vi "核查数据发送(子VI).vi"(8 "错误输入":errorcluster) -> (0 "错误输出":errorcluster)   [LabVIEW 2016, in "数据传输系统.lvlib"]
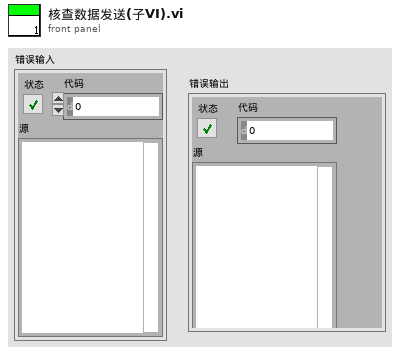
[diagram p1: front panel]
types:
  T1 = enum16{"质控数据", "操作日志", "仪器参数", "系统状态", "运行模式", "测量周期", "超标留样", "报警信息", "环境参数"}
  T2 = enum16{"空白测试", "跨度核查", "标样核查", "加标回收", "平行样", "集成干预"}
  T3 = cluster{"氨氮零点核查索引起始时间":string, "总磷零点核查索引起始时间":string, "总氮零点核查索引起始时间":string, "CODMn零点核查索引起始时间":string, "CODCr零点核查索引起始时间":string, "亚硝酸盐零点核查索引起始时间":string, "硫化物零点核查索引起始时间":string, "ORP零点核查索引起始时间":string}
  T4 = cluster{"[0]":string, "[1]":string, "[2]":string, "[3]":string, "[4]":string, "[5]":string, "[6]":string, "[7]":string}
  T5 = cluster{"PH":string[][], "CODCr":string[][], "氨氮":string[][], "CODMn":string[][], "总氮":string[][], "总磷":string[][], "电导率":string[][], "水温":string[][], "DO":string[][], "浊度":string[][], "叶绿素":string[][], "藻密度":string[][], "铜":string[][], "盐度":string[][], "水位":string[][], "流速":string[][], "瞬时流量":string[][], "累积流量":string[][], "亚硝酸盐":string[][], "硫化物":string[][], "ORP":string[][], "铅":string[][], "镉":string[][], "锌":string[][], "镍":string[][], "锰":string[][], "汞":string[][], "气温":string[][], "气压":string[][], "风速":string[][], "风向":string[][]}
  T6 = cluster{"氨氮跨度核查索引起始时间":string, "总磷跨度核查索引起始时间":string, "总氮跨度核查索引起始时间":string, "CODMn跨度核查索引起始时间":string, "CODCr跨度核查索引起始时间":string, "亚硝酸盐跨度核查索引起始时间":string, "硫化物跨度核查索引起始时间":string, "ORP跨度核查索引起始时间":string}
  T7 = cluster{"氨氮标样核查索引起始时间":string, "总磷标样核查索引起始时间":string, "总氮标样核查索引起始时间":string, "CODMn标样核查索引起始时间":string, "CODCr标样核查索引起始时间":string, "DO标样核查索引起始时间":string, "PH标样核查索引起始时间":string, "比电导率标样核查索引起始时间":string, "水温标样核查索引起始时间":string, "浊度标样核查索引起始时间":string, "叶绿素a标样核查索引起始时间":string, "藻密度标样核查索引起始时间":string, "亚硝酸盐标样核查索引起始时间":string, "硫化物标样核查索引起始时间":string, "ORP标样核查索引起始时间":string}
  T8 = cluster{"[0]":string, "[1]":string, "[2]":string, "[3]":string, "[4]":string, "[5]":string, "[6]":string, "[7]":string, "[8]":string, "[9]":string, "[10]":string, "[11]":string, "[12]":string, "[13]":string, "[14]":string}
  T9 = cluster{"氨氮加标回收索引起始时间":string, "总磷加标回收索引起始时间":string, "总氮加标回收索引起始时间":string, "CODMn加标回收索引起始时间":string, "CODCr加标回收索引起始时间":string}
  T10 = cluster{"[0]":string, "[1]":string, "[2]":string, "[3]":string, "[4]":string}
  T11 = cluster{"氨氮平行样索引起始时间":string, "总磷平行样索引起始时间":string, "总氮平行样索引起始时间":string, "CODMn平行样索引起始时间":string, "CODCr平行样索引起始时间":string}
  T12 = cluster{"氨氮集成干预索引起始时间":string, "总磷集成干预索引起始时间":string, "总氮集成干预索引起始时间":string, "CODMn集成干预索引起始时间":string, "CODCr集成干预索引起始时间":string, "DO集成干预索引起始时间":string, "PH集成干预索引起始时间":string, "比电导率集成干预索引起始时间":string, "水温集成干预索引起始时间":string, "浊度集成干预索引起始时间":string, "叶绿素a集成干预索引起始时间":string, "藻密度集成干预索引起始时间":string, "亚硝酸盐集成干预索引起始时间":string, "硫化物集成干预索引起始时间":string, "ORP集成干预索引起始时间":string}
  T13 = cluster{"氨氮仪器日志索引起始时间":string, "总磷仪器日志索引起始时间":string, "总氮仪器日志索引起始时间":string, "CODMn仪器日志索引起始时间":string, "CODCr仪器日志索引起始时间":string, "系统仪器日志索引起始时间":string}
  T14 = cluster{"[0]":string, "[1]":string, "[2]":string, "[3]":string, "[4]":string, "[5]":string}
  T15 = cluster{"氨氮仪器参数索引起始时间":string, "总磷仪器参数索引起始时间":string, "总氮仪器参数索引起始时间":string, "CODMn仪器参数索引起始时间":string, "CODCr仪器参数索引起始时间":string, "DO仪器参数索引起始时间":string, "PH仪器参数索引起始时间":string, "比电导率仪器参数索引起始时间":string, "水温仪器参数索引起始时间":string, "浊度仪器参数索引起始时间":string, "叶绿素a仪器参数索引起始时间":string, "藻密度仪器参数索引起始时间":string, "ORP仪器参数索引起始时间":string}
  T16 = cluster{"[0]":string, "[1]":string, "[2]":string, "[3]":string, "[4]":string, "[5]":string, "[6]":string, "[7]":string, "[8]":string, "[9]":string, "[10]":string, "[11]":string, "[12]":string}
  T17 = cluster{"氨氮报警信息索引起始时间":string, "总磷报警信息索引起始时间":string, "总氮报警信息索引起始时间":string, "CODMn报警信息索引起始时间":string, "CODCr报警信息索引起始时间":string, "DO报警信息索引起始时间":string, "PH报警信息索引起始时间":string, "比电导率报警信息索引起始时间":string, "水温报警信息索引起始时间":string, "浊度报警信息索引起始时间":string, "叶绿素报警信息索引起始时间":string, "系统报警信息索引起始时间":string}
  T18 = cluster{"[0]":string, "[1]":string, "[2]":string, "[3]":string, "[4]":string, "[5]":string, "[6]":string, "[7]":string, "[8]":string, "[9]":string, "[10]":string, "[11]":string}
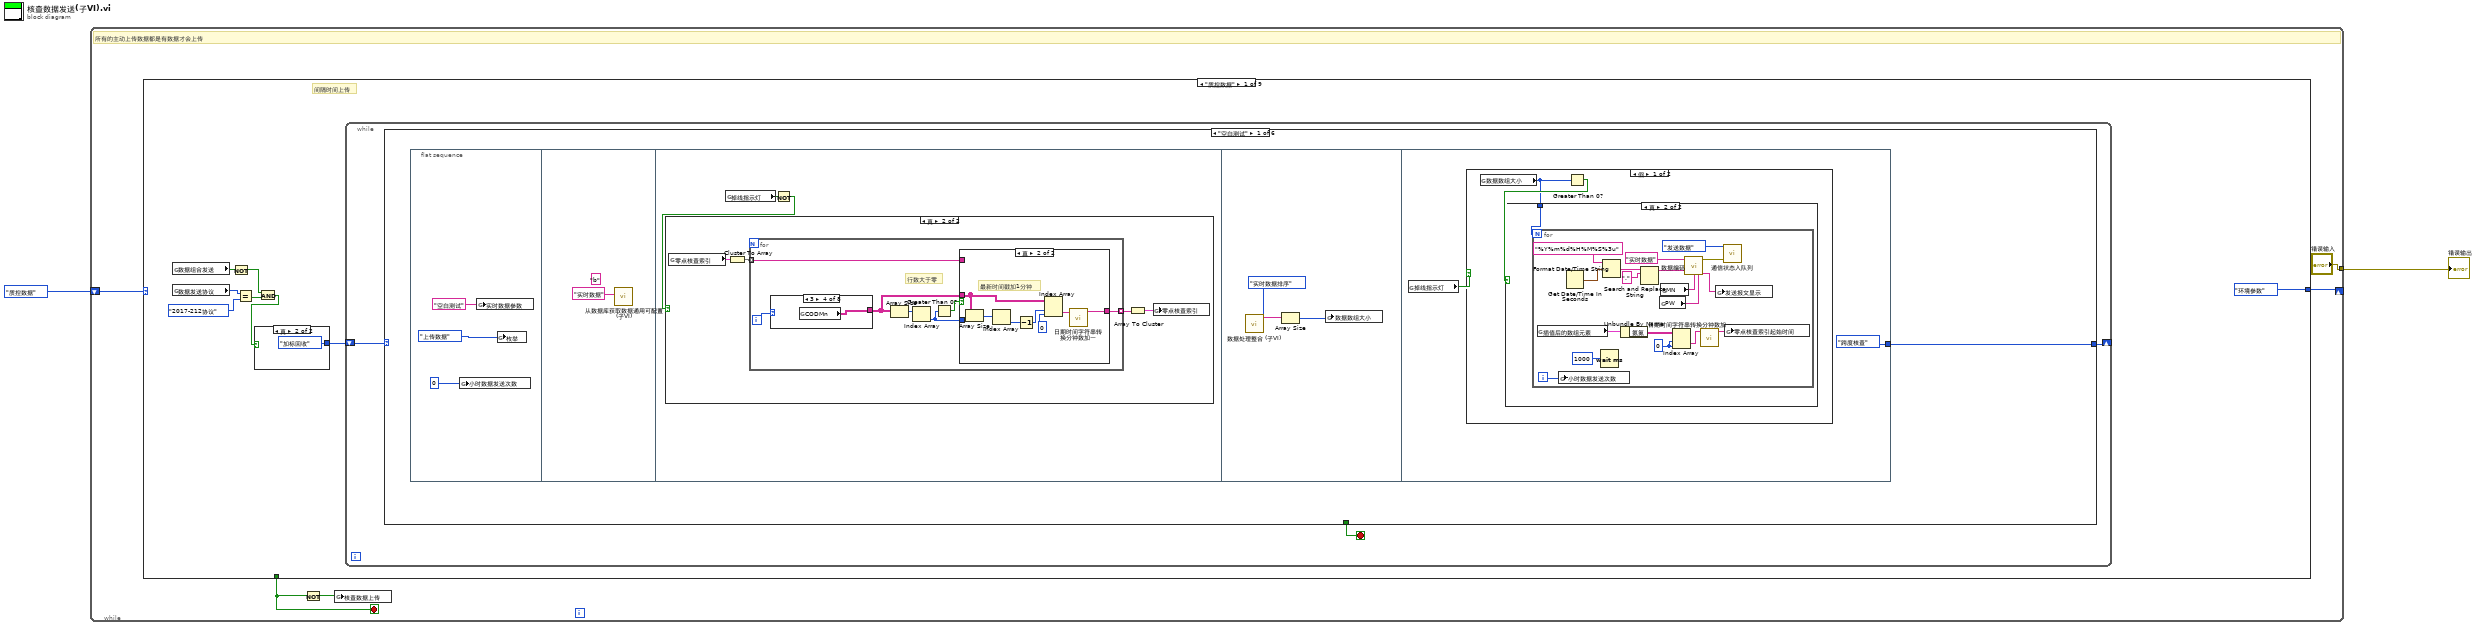
[diagram p0: block diagram]
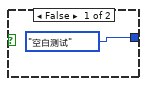
[diagram p2: hidden frame]
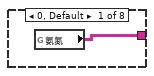
[diagram p4: hidden frame]
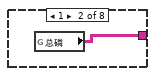
[diagram p5: hidden frame]
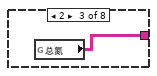
[diagram p6: hidden frame]
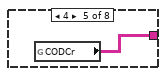
[diagram p7: hidden frame]
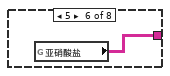
[diagram p8: hidden frame]
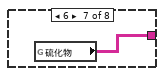
[diagram p9: hidden frame]
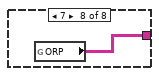
[diagram p10: hidden frame]
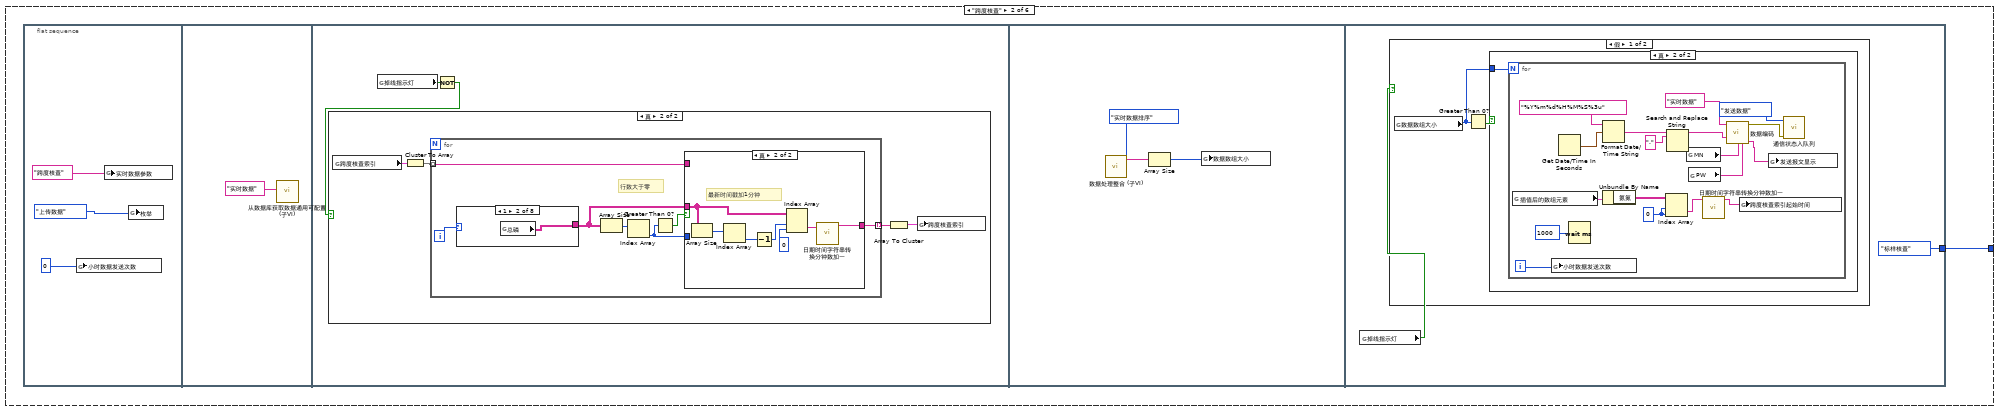
[diagram p14: hidden frame]
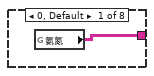
[diagram p16: hidden frame]
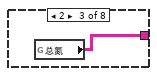
[diagram p17: hidden frame]
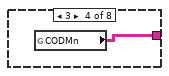
[diagram p18: hidden frame]
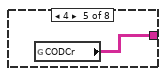
[diagram p19: hidden frame]
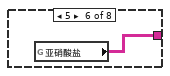
[diagram p20: hidden frame]
diagram:
  n1 = while "While循环" {
    shift-right: [w6] -> _
    shift-left: T1."质控数据" -> [w7]
    tunnel: ["错误输入"] -> w1
    stop <- w4 stop-if-true
    # "所有的主动上传数据都是有数据才会上传"
    n2 = case shown="\"质控数据\"" w7 {
      tunnel: [T1."环境参数" T1."仪器参数" T1."系统状态" T1."运行模式" T1."测量周期" T1."超标留样" T1."报警信息" T1."环境参数" T1."环境参数"] -> w6
      tunnel: [_ _ _ _ _ _ _ _ TRUE] -> w4
      frame "质控数据" {
        # "间隔时间上传"
        n3 = global read "断电保存全局.vi" "数据组合发送"() -> (w10:bool)
        n4 = global read "断电保存全局.vi" "数据发送协议"() -> (w13:enum16{"2005-212协议", "2017-212协议"})
        n5 = Not(x=w10) -> (.not. x?=w9:bool)
        n6 = Equal?(x=w13, y=enum16{"2005-212协议", "2017-212协议"}."2017-212协议" ("数据发送协议")) -> (x = y?=w11:bool)
        n7 = And(x=w9, y=w11) -> (x .and. y?=w8:bool)
        n8 = case shown="真" w8 {
          tunnel: [T2."空白测试" T2."加标回收"] -> w15
          frame False {
          }
          frame True {
          }
        }
        n9 = while {
          shift-right: [w18] -> _
          shift-left: w15 -> [w19]
          stop <- w20 stop-if-true
          n10 = case shown="\"空白测试\"" w19 {
            tunnel: [_ _ _ _ _ TRUE] -> w20
            tunnel: [w21 w81 w141 w208 w267 w319] -> w18
            frame "空白测试" {
              n11 = flat-sequence {
                tunnel: [T2."跨度核查"] -> w21
                frame #0 {
                  n12 = global write "全局 小时数据发送次数.vi" "小时数据发送次数"(0 ("小时数据发送次数")) -> ()
                  n13 = global write "全局 实时数据参数.vi" "实时数据参数"("空白测试") -> ()
                  n14 = global write "全局1.vi" "枚举"(enum16{"返回请求应答", "上传数据", "返回执行结果"}."上传数据" ("枚举")) -> ()
                }
                frame #1 {
                  (unwired) "b" ("列队名（唯一）")
                  n15 = call "从数据库获取数据通用可配置(子VI).vi"("table输入"="实时数据" ("新元素/子数组")) -> ()  [unwired: 9 in, 2 out]
                }
                frame #2 {
                  n16 = global read "全局 数据发送重叠.vi" "掉线指示灯"() -> (w27:bool)
                  n17 = Not(x=w27) -> (.not. x?=w26:bool)
                  n18 = case shown="真" w26 {
                    frame False {
                    }
                    frame True {
                      n19 = global read "全局 时间2.vi" "零点核查索引"() -> (w31:T3)
                      n20 = Cluster To Array(cluster=w31) -> (array=w30:string[])
                      n21 = for {
                        tunnel: [w33] -> w29 mode=indexing
                        tunnel: w30 -> [w32] mode=indexing
                        i -> [w34]
                        # "行数大于零"
                        n22 = case shown="3" w34 {
                          tunnel: [w39 w40 w41 w42 w43 w44 w45 w46] -> w35
                          frame 0, Default {
                            n23 = global read "全局 所有参数.vi" "氨氮"() -> (w39:string[][])
                          }
                          frame 1 {
                            n24 = global read "全局 所有参数.vi" "总磷"() -> (w40:string[][])
                          }
                          frame 2 {
                            n25 = global read "全局 所有参数.vi" "总氮"() -> (w41:string[][])
                          }
                          frame 3 {
                            n26 = global read "全局 所有参数.vi" "CODMn"() -> (w42:string[][])
                          }
                          frame 4 {
                            n27 = global read "全局 所有参数.vi" "CODCr"() -> (w43:string[][])
                          }
                          frame 5 {
                            n28 = global read "全局 所有参数.vi" "亚硝酸盐"() -> (w44:string[][])
                          }
                          frame 6 {
                            n29 = global read "全局 所有参数.vi" "硫化物"() -> (w45:string[][])
                          }
                          frame 7 {
                            n30 = global read "全局 所有参数.vi" "ORP"() -> (w46:string[][])
                          }
                        }
                        n31 = Array Size(array=w35) -> (size(s)=w37:i32[])
                        n32 = Index Array(array=w37) -> (element=w36:i32)  [unwired: 1 in]
                        n33 = Greater Than 0?(x=w36) -> (x > 0?=w38:bool)
                        n34 = case shown="真" w38 {
                          tunnel: w36 -> [_ _]
                          tunnel: w35 -> [_ w50]
                          tunnel: [w47 w48] -> w33
                          tunnel: w32 -> [w47 _]
                          frame False {
                          }
                          frame True {
                            # "最新时间戳加1分钟"
                            n35 = Array Size(array=w50) -> (size(s)=w53:i32[])
                            n36 = Index Array(array=w53) -> (element=w52:i32)  [unwired: 1 in]
                            n37 = Decrement(x=w52) -> (x-1=w51:i32)
                            n38 = Index Array(array=w50, index (row)=w51, index (col)=0 ("禁用的索引 (列)")) -> (element=w54:string)
                            n39 = call "日期时间字符串转换分钟数加一.vi"("data[0]"=w54) -> ("日期/时间字符串"=w48:string)  [unwired: 10 in]
                          }
                        }
                      }
                      n40 = Array To Cluster(array=w29) -> (cluster=w28:T4)
                      n41 = global write "全局 时间2.vi" "零点核查索引"(w28) -> ()
                    }
                  }
                }
                frame #3 {
                  n42 = call "数据处理整合 (子VI).vi"("枚举"=enum16{"实时数据排序", "小时数据排序"}."实时数据排序") -> ("已排序的数组"=w57:string[])  [unwired: 10 in]
                  n43 = Array Size(array=w57) -> (size(s)=w56:i32)
                  n44 = global write "全局 数据数组大小.vi" "数据数组大小"(w56) -> ()
                }
                frame #4 {
                  n45 = global read "全局 数据发送重叠.vi" "掉线指示灯"() -> (w59:bool)
                  n46 = case shown="假" w59 {
                    frame False {
                      n47 = global read "全局 数据数组大小.vi" "数据数组大小"() -> (w60:i32)
                      n48 = Greater Than 0?(x=w60) -> (x > 0?=w61:bool)
                      n49 = case shown="真" w61 {
                        tunnel: w60 -> [_ w62]
                        frame False {
                        }
                        frame True {
                          n50 = for {
                            N: w62 -> [_]
                            i -> [w63]
                            w75 = 0 ("禁用的索引 (列)")
                            n51 = global read "插值后的新数组.vi" "插值后的数组元素"() -> (w79:T5)
                            n52 = global write "全局 小时数据发送次数.vi" "小时数据发送次数"(w63) -> ()
                            n53 = Get Date/Time In Seconds() -> (seconds since 1Jan1904=w67:timestamp)
                            n54 = Wait (ms)(milliseconds to wait=u32 1000 ("等待时间（毫秒）")) -> ()  [unwired: 1 out]
                            n55 = Format Date/Time String(time format string (%c)="%Y%m%d%H%M%S%3u" ("时间格式字符串(%c)"), seconds (now)=w67) -> (date/time string=w66:string)  [unwired: 1 in]
                            n56 = Unbundle By Name(w79) -> ("氨氮"=w78:string[][])
                            n57 = Search and Replace String(input string=w66, search string="." ("搜索字符串")) -> (result string=w64:string)  [unwired: 6 in, 3 out]
                            n58 = global read "断电保存全局.vi" "PW"() -> (w71:string)
                            n59 = global read "断电保存全局.vi" "MN"() -> (w72:string)
                            n60 = Index Array(array=w78, index (row)=w75, index (col)=w75) -> (element=w77:string)
                            n61 = call "数据编码.vi"("table输入"="实时数据" ("新元素/子数组"), "QN"=w64, "MN"=w72, "PW"=w71) -> ("错误常量"=w70:errorcluster, "通讯包字符串"=w74:string)  [unwired: 10 in]
                            n62 = call "日期时间字符串转换分钟数加一.vi"("data[0]"=w77) -> ("日期/时间字符串"=w76:string)  [unwired: 10 in]
                            n63 = global write "全局1.vi" "发送报文显示"(w74) -> ()
                            n64 = call "通信状态入队列.vi"("错误输入（无错误）"=w70, "枚举"=enum16{"打开连接", "发送数据", "读取数据", "数据处理", "关闭连接"}."发送数据") -> ()  [unwired: 9 in, 1 out]
                            n65 = global write "全局 时间2.vi" "零点核查索引起始时间"(w76) -> ()
                          }
                        }
                      }
                    }
                    frame True {
                    }
                  }
                }
              }
            }
            frame "跨度核查" {
              n66 = flat-sequence {
                tunnel: [T2."标样核查"] -> w81
                frame #0 {
                  n67 = global write "全局 小时数据发送次数.vi" "小时数据发送次数"(0 ("小时数据发送次数")) -> ()
                  n68 = global write "全局 实时数据参数.vi" "实时数据参数"("跨度核查") -> ()
                  n69 = global write "全局1.vi" "枚举"(enum16{"返回请求应答", "上传数据", "返回执行结果"}."上传数据" ("枚举")) -> ()
                }
                frame #1 {
                  n70 = call "从数据库获取数据通用可配置(子VI).vi"("table输入"="实时数据" ("新元素/子数组")) -> ()  [unwired: 9 in, 2 out]
                }
                frame #2 {
                  n71 = global read "全局 数据发送重叠.vi" "掉线指示灯"() -> (w87:bool)
                  n72 = Not(x=w87) -> (.not. x?=w86:bool)
                  n73 = case shown="真" w86 {
                    frame False {
                    }
                    frame True {
                      n74 = global read "全局 时间2.vi" "跨度核查索引"() -> (w91:T6)
                      n75 = Cluster To Array(cluster=w91) -> (array=w90:string[])
                      n76 = for {
                        tunnel: [w93] -> w89 mode=indexing
                        tunnel: w90 -> [w92] mode=indexing
                        i -> [w94]
                        # "行数大于零"
                        n77 = case shown="1" w94 {
                          tunnel: [w99 w100 w101 w102 w103 w104 w105 w106] -> w95
                          frame 0, Default {
                            n78 = global read "全局 所有参数.vi" "氨氮"() -> (w99:string[][])
                          }
                          frame 1 {
                            n79 = global read "全局 所有参数.vi" "总磷"() -> (w100:string[][])
                          }
                          frame 2 {
                            n80 = global read "全局 所有参数.vi" "总氮"() -> (w101:string[][])
                          }
                          frame 3 {
                            n81 = global read "全局 所有参数.vi" "CODMn"() -> (w102:string[][])
                          }
                          frame 4 {
                            n82 = global read "全局 所有参数.vi" "CODCr"() -> (w103:string[][])
                          }
                          frame 5 {
                            n83 = global read "全局 所有参数.vi" "亚硝酸盐"() -> (w104:string[][])
                          }
                          frame 6 {
                            n84 = global read "全局 所有参数.vi" "硫化物"() -> (w105:string[][])
                          }
                          frame 7 {
                            n85 = global read "全局 所有参数.vi" "ORP"() -> (w106:string[][])
                          }
                        }
                        n86 = Array Size(array=w95) -> (size(s)=w97:i32[])
                        n87 = Index Array(array=w97) -> (element=w96:i32)  [unwired: 1 in]
                        n88 = Greater Than 0?(x=w96) -> (x > 0?=w98:bool)
                        n89 = case shown="真" w98 {
                          tunnel: w96 -> [_ _]
                          tunnel: w95 -> [_ w110]
                          tunnel: [w107 w108] -> w93
                          tunnel: w92 -> [w107 _]
                          frame False {
                          }
                          frame True {
                            # "最新时间戳加1分钟"
                            n90 = Array Size(array=w110) -> (size(s)=w113:i32[])
                            n91 = Index Array(array=w113) -> (element=w112:i32)  [unwired: 1 in]
                            n92 = Decrement(x=w112) -> (x-1=w111:i32)
                            n93 = Index Array(array=w110, index (row)=w111, index (col)=0 ("禁用的索引 (列)")) -> (element=w114:string)
                            n94 = call "日期时间字符串转换分钟数加一.vi"("data[0]"=w114) -> ("日期/时间字符串"=w108:string)  [unwired: 10 in]
                          }
                        }
                      }
                      n95 = Array To Cluster(array=w89) -> (cluster=w88:T4)
                      n96 = global write "全局 时间2.vi" "跨度核查索引"(w88) -> ()
                    }
                  }
                }
                frame #3 {
                  n97 = call "数据处理整合 (子VI).vi"("枚举"=enum16{"实时数据排序", "小时数据排序"}."实时数据排序") -> ("已排序的数组"=w117:string[])  [unwired: 10 in]
                  n98 = Array Size(array=w117) -> (size(s)=w116:i32)
                  n99 = global write "全局 数据数组大小.vi" "数据数组大小"(w116) -> ()
                }
                frame #4 {
                  n100 = global read "全局 数据发送重叠.vi" "掉线指示灯"() -> (w119:bool)
                  n101 = case shown="假" w119 {
                    frame False {
                      n102 = global read "全局 数据数组大小.vi" "数据数组大小"() -> (w120:i32)
                      n103 = Greater Than 0?(x=w120) -> (x > 0?=w121:bool)
                      n104 = case shown="真" w121 {
                        tunnel: w120 -> [_ w122]
                        frame False {
                        }
                        frame True {
                          n105 = for {
                            N: w122 -> [_]
                            i -> [w123]
                            w135 = 0 ("禁用的索引 (列)")
                            n106 = global read "插值后的新数组.vi" "插值后的数组元素"() -> (w139:T5)
                            n107 = global write "全局 小时数据发送次数.vi" "小时数据发送次数"(w123) -> ()
                            n108 = Get Date/Time In Seconds() -> (seconds since 1Jan1904=w127:timestamp)
                            n109 = Wait (ms)(milliseconds to wait=u32 1000 ("等待时间（毫秒）")) -> ()  [unwired: 1 out]
                            n110 = Format Date/Time String(time format string (%c)="%Y%m%d%H%M%S%3u" ("时间格式字符串(%c)"), seconds (now)=w127) -> (date/time string=w126:string)  [unwired: 1 in]
                            n111 = Unbundle By Name(w139) -> ("氨氮"=w138:string[][])
                            n112 = Index Array(array=w138, index (row)=w135, index (col)=w135) -> (element=w137:string)
                            n113 = Search and Replace String(input string=w126, search string="." ("搜索字符串")) -> (result string=w124:string)  [unwired: 6 in, 3 out]
                            n114 = global read "断电保存全局.vi" "MN"() -> (w133:string)
                            n115 = global read "断电保存全局.vi" "PW"() -> (w132:string)
                            n116 = call "日期时间字符串转换分钟数加一.vi"("data[0]"=w137) -> ("日期/时间字符串"=w136:string)  [unwired: 10 in]
                            n117 = call "数据编码.vi"("table输入"="实时数据" ("新元素/子数组"), "QN"=w124, "MN"=w133, "PW"=w132) -> ("错误常量"=w130:errorcluster, "通讯包字符串"=w131:string)  [unwired: 10 in]
                            n118 = global write "全局 时间2.vi" "跨度核查索引起始时间"(w136) -> ()
                            n119 = global write "全局1.vi" "发送报文显示"(w131) -> ()
                            n120 = call "通信状态入队列.vi"("错误输入（无错误）"=w130, "枚举"=enum16{"打开连接", "发送数据", "读取数据", "数据处理", "关闭连接"}."发送数据") -> ()  [unwired: 9 in, 1 out]
                          }
                        }
                      }
                    }
                    frame True {
                    }
                  }
                }
              }
            }
            frame "标样核查" {
              n121 = flat-sequence {
                tunnel: [T2."加标回收"] -> w141
                frame #0 {
                  n122 = global write "全局 小时数据发送次数.vi" "小时数据发送次数"(0 ("小时数据发送次数")) -> ()
                  n123 = global write "全局 实时数据参数.vi" "实时数据参数"("核查数据") -> ()
                  n124 = global write "全局1.vi" "枚举"(enum16{"返回请求应答", "上传数据", "返回执行结果"}."上传数据" ("枚举")) -> ()
                }
                frame #1 {
                  (unwired) "n" ("列队名（唯一）")
                  n125 = call "从数据库获取数据通用可配置(子VI).vi"("table输入"="实时数据" ("新元素/子数组")) -> ()  [unwired: 9 in, 2 out]
                }
                frame #2 {
                  n126 = global read "全局 数据发送重叠.vi" "掉线指示灯"() -> (w147:bool)
                  n127 = Not(x=w147) -> (.not. x?=w146:bool)
                  n128 = case shown="真" w146 {
                    frame False {
                    }
                    frame True {
                      n129 = global read "全局 时间2.vi" "标样核查索引"() -> (w151:T7)
                      n130 = Cluster To Array(cluster=w151) -> (array=w150:string[])
                      n131 = for {
                        tunnel: [w153] -> w148 mode=indexing
                        tunnel: w150 -> [w152] mode=indexing
                        i -> [w154]
                        # "行数大于零"
                        n132 = case shown="0, 默认" w154 {
                          tunnel: [w159 w160 w161 w162 w163 w164 w165 w166 w167 w168 w169 w170 w171 w172 w173] -> w155
                          frame 0, Default {
                            n133 = global read "全局 所有参数.vi" "氨氮"() -> (w159:string[][])
                          }
                          frame 1 {
                            n134 = global read "全局 所有参数.vi" "总磷"() -> (w160:string[][])
                          }
                          frame 2 {
                            n135 = global read "全局 所有参数.vi" "总氮"() -> (w161:string[][])
                          }
                          frame 3 {
                            n136 = global read "全局 所有参数.vi" "CODMn"() -> (w162:string[][])
                          }
                          frame 4 {
                            n137 = global read "全局 所有参数.vi" "CODCr"() -> (w163:string[][])
                          }
                          frame 5 {
                            n138 = global read "全局 所有参数.vi" "DO"() -> (w164:string[][])
                          }
                          frame 6 {
                            n139 = global read "全局 所有参数.vi" "PH"() -> (w165:string[][])
                          }
                          frame 7 {
                            n140 = global read "全局 所有参数.vi" "电导率"() -> (w166:string[][])
                          }
                          frame 8 {
                            n141 = global read "全局 所有参数.vi" "水温"() -> (w167:string[][])
                          }
                          frame 9 {
                            n142 = global read "全局 所有参数.vi" "浊度"() -> (w168:string[][])
                          }
                          frame 10 {
                            n143 = global read "全局 所有参数.vi" "叶绿素"() -> (w169:string[][])
                          }
                          frame 11 {
                            n144 = global read "全局 所有参数.vi" "藻密度"() -> (w170:string[][])
                          }
                          frame 12 {
                            n145 = global read "全局 所有参数.vi" "亚硝酸盐"() -> (w171:string[][])
                          }
                          frame 13 {
                            n146 = global read "全局 所有参数.vi" "硫化物"() -> (w172:string[][])
                          }
                          frame 14 {
                            n147 = global read "全局 所有参数.vi" "ORP"() -> (w173:string[][])
                          }
                        }
                        n148 = Array Size(array=w155) -> (size(s)=w157:i32[])
                        n149 = Index Array(array=w157) -> (element=w156:i32)  [unwired: 1 in]
                        n150 = Greater Than 0?(x=w156) -> (x > 0?=w158:bool)
                        n151 = case shown="真" w158 {
                          tunnel: w154 -> [_ _]
                          tunnel: w156 -> [_ _]
                          tunnel: w155 -> [_ w176]
                          tunnel: [w174 w175] -> w153
                          tunnel: w152 -> [w174 _]
                          frame False {
                          }
                          frame True {
                            # "最新时间戳加1分钟"
                            n152 = Array Size(array=w176) -> (size(s)=w180:i32[])
                            n153 = Index Array(array=w180) -> (element=w179:i32)  [unwired: 1 in]
                            n154 = Decrement(x=w179) -> (x-1=w178:i32)
                            n155 = Index Array(array=w176, index (row)=w178, index (col)=0 ("禁用的索引 (列)")) -> (element=w181:string)
                            n156 = call "日期时间字符串转换分钟数加一.vi"("data[0]"=w181) -> ("日期/时间字符串"=w175:string)  [unwired: 10 in]
                          }
                        }
                      }
                      n157 = Array To Cluster(array=w148) -> (cluster=w149:T8)
                      n158 = global write "全局 时间2.vi" "标样核查索引"(w149) -> ()
                    }
                  }
                }
                frame #3 {
                  n159 = call "数据处理整合 (子VI).vi"("枚举"=enum16{"实时数据排序", "小时数据排序"}."实时数据排序") -> ("已排序的数组"=w184:string[])  [unwired: 10 in]
                  n160 = Array Size(array=w184) -> (size(s)=w183:i32)
                  n161 = global write "全局 数据数组大小.vi" "数据数组大小"(w183) -> ()
                }
                frame #4 {
                  n162 = global read "全局 数据发送重叠.vi" "掉线指示灯"() -> (w186:bool)
                  n163 = case shown="假" w186 {
                    frame False {
                      n164 = global read "全局 数据数组大小.vi" "数据数组大小"() -> (w187:i32)
                      n165 = Greater Than 0?(x=w187) -> (x > 0?=w188:bool)
                      n166 = case shown="真" w188 {
                        tunnel: w187 -> [_ w189]
                        frame False {
                        }
                        frame True {
                          n167 = for {
                            N: w189 -> [_]
                            i -> [w190]
                            w202 = 0 ("禁用的索引 (列)")
                            n168 = global read "插值后的新数组.vi" "插值后的数组元素"() -> (w206:T5)
                            n169 = Get Date/Time In Seconds() -> (seconds since 1Jan1904=w194:timestamp)
                            n170 = Wait (ms)(milliseconds to wait=u32 1000 ("等待时间（毫秒）")) -> ()  [unwired: 1 out]
                            n171 = Format Date/Time String(time format string (%c)="%Y%m%d%H%M%S%3u" ("时间格式字符串(%c)"), seconds (now)=w194) -> (date/time string=w193:string)  [unwired: 1 in]
                            n172 = Unbundle By Name(w206) -> ("氨氮"=w205:string[][])
                            n173 = global write "全局 小时数据发送次数.vi" "小时数据发送次数"(w190) -> ()
                            n174 = global read "断电保存全局.vi" "MN"() -> (w199:string)
                            n175 = Search and Replace String(input string=w193, search string="." ("搜索字符串")) -> (result string=w191:string)  [unwired: 6 in, 3 out]
                            n176 = global read "断电保存全局.vi" "PW"() -> (w198:string)
                            n177 = Index Array(array=w205, index (row)=w202, index (col)=w202) -> (element=w204:string)
                            n178 = call "日期时间字符串转换分钟数加一.vi"("data[0]"=w204) -> ("日期/时间字符串"=w203:string)  [unwired: 10 in]
                            n179 = call "数据编码.vi"("table输入"="实时数据" ("新元素/子数组"), "QN"=w191, "MN"=w199, "PW"=w198) -> ("错误常量"=w197:errorcluster, "通讯包字符串"=w201:string)  [unwired: 10 in]
                            n180 = global write "全局 时间2.vi" "标样核查索引起始时间"(w203) -> ()
                            n181 = global write "全局1.vi" "发送报文显示"(w201) -> ()
                            n182 = call "通信状态入队列.vi"("错误输入（无错误）"=w197, "枚举"=enum16{"打开连接", "发送数据", "读取数据", "数据处理", "关闭连接"}."发送数据") -> ()  [unwired: 9 in, 1 out]
                          }
                        }
                      }
                    }
                    frame True {
                    }
                  }
                }
              }
            }
            frame "加标回收" {
              n183 = flat-sequence {
                tunnel: [T2."平行样"] -> w208
                frame #0 {
                  n184 = global write "全局 小时数据发送次数.vi" "小时数据发送次数"(0 ("小时数据发送次数")) -> ()
                  n185 = global write "全局 实时数据参数.vi" "实时数据参数"("加标回收测试") -> ()
                  n186 = global write "全局1.vi" "枚举"(enum16{"返回请求应答", "上传数据", "返回执行结果"}."上传数据" ("枚举")) -> ()
                }
                frame #1 {
                  (unwired) "d" ("列队名（唯一）")
                  n187 = call "从数据库获取数据通用可配置(子VI).vi"("table输入"="加标回收" ("新元素/子数组")) -> ()  [unwired: 9 in, 2 out]
                }
                frame #2 {
                  n188 = global read "全局 数据发送重叠.vi" "掉线指示灯"() -> (w214:bool)
                  n189 = Not(x=w214) -> (.not. x?=w213:bool)
                  n190 = case shown="真" w213 {
                    frame False {
                    }
                    frame True {
                      n191 = global read "全局 时间2.vi" "加标回收索引"() -> (w218:T9)
                      n192 = Cluster To Array(cluster=w218) -> (array=w217:string[])
                      n193 = for {
                        tunnel: [w220] -> w215 mode=indexing
                        tunnel: w217 -> [w219] mode=indexing
                        i -> [w221]
                        # "行数大于零"
                        n194 = case shown="0, 默认" w221 {
                          tunnel: [w226 w227 w228 w229 w230] -> w222
                          frame 0, Default {
                            n195 = global read "全局 所有参数.vi" "氨氮加标回收率"() -> (w226:string[][])
                          }
                          frame 1 {
                            n196 = global read "全局 所有参数.vi" "总磷加标回收率"() -> (w227:string[][])
                          }
                          frame 2 {
                            n197 = global read "全局 所有参数.vi" "总氮加标回收率"() -> (w228:string[][])
                          }
                          frame 3 {
                            n198 = global read "全局 所有参数.vi" "CODMn加标回收率"() -> (w229:string[][])
                          }
                          frame 4 {
                            n199 = global read "全局 所有参数.vi" "CODCr加标回收率"() -> (w230:string[][])
                          }
                        }
                        n200 = Array Size(array=w222) -> (size(s)=w224:i32[])
                        n201 = Index Array(array=w224) -> (element=w223:i32)  [unwired: 1 in]
                        n202 = Greater Than 0?(x=w223) -> (x > 0?=w225:bool)
                        n203 = case shown="真" w225 {
                          tunnel: w221 -> [_ _]
                          tunnel: w223 -> [_ _]
                          tunnel: w222 -> [_ w235]
                          tunnel: [w231 w232] -> w220
                          tunnel: w219 -> [w231 _]
                          frame False {
                          }
                          frame True {
                            # "最新时间戳加1分钟"
                            n204 = Array Size(array=w235) -> (size(s)=w237:i32[])
                            n205 = Index Array(array=w237) -> (element=w236:i32)  [unwired: 1 in]
                            n206 = Decrement(x=w236) -> (x-1=w234:i32)
                            n207 = Index Array(array=w235, index (row)=w234, index (col)=0 ("禁用的索引 (列)")) -> (element=w238:string)
                            n208 = call "日期时间字符串转换分钟数加一.vi"("data[0]"=w238) -> ("日期/时间字符串"=w232:string)  [unwired: 10 in]
                          }
                        }
                      }
                      n209 = Array To Cluster(array=w215) -> (cluster=w216:T10)
                      n210 = global write "全局 时间2.vi" "加标回收索引"(w216) -> ()
                    }
                  }
                }
                frame #3 {
                  n211 = call "加标回收数据处理整合 (子VI).vi"("枚举"=enum16{"实时数据排序", "小时数据排序"}."实时数据排序") -> ("已排序的数组"=w240:string[])  [unwired: 10 in]
                  n212 = Array Size(array=w240) -> (size(s)=w241:i32)
                  n213 = global write "全局 数据数组大小.vi" "数据数组大小"(w241) -> ()
                }
                frame #4 {
                  n214 = global read "全局 数据发送重叠.vi" "掉线指示灯"() -> (w243:bool)
                  n215 = case shown="假" w243 {
                    frame False {
                      n216 = global read "全局 数据数组大小.vi" "数据数组大小"() -> (w244:i32)
                      n217 = Greater Than 0?(x=w244) -> (x > 0?=w245:bool)
                      n218 = case shown="真" w245 {
                        tunnel: w244 -> [_ w246]
                        frame False {
                        }
                        frame True {
                          n219 = for {
                            N: w246 -> [_]
                            i -> [w247]
                            n220 = global read "全局 数据数组大小.vi" "数据数组大小"() -> (w262:i32)
                            n221 = global read "插值后的新数组.vi" "插值后的数组元素"() -> (w265:T5)
                            n222 = Get Date/Time In Seconds() -> (seconds since 1Jan1904=w251:timestamp)
                            n223 = Format Date/Time String(time format string (%c)="%Y%m%d%H%M%S%3u" ("时间格式字符串(%c)"), seconds (now)=w251) -> (date/time string=w250:string)  [unwired: 1 in]
                            n224 = Decrement(x=w262) -> (x-1=w261:i32)
                            n225 = Unbundle By Name(w265) -> ("氨氮"=w264:string[][])
                            n226 = Search and Replace String(input string=w250, search string="." ("搜索字符串")) -> (result string=w248:string)  [unwired: 6 in, 3 out]
                            n227 = global write "全局 小时数据发送次数.vi" "小时数据发送次数"(w247) -> ()
                            n228 = global read "断电保存全局.vi" "MN"() -> (w256:string)
                            n229 = Index Array(array=w264, index (row)=w261, index (col)=0 ("禁用的索引 (列)")) -> (element=w260:string)
                            n230 = global read "断电保存全局.vi" "PW"() -> (w255:string)
                            n231 = call "日期时间字符串转换分钟数加一.vi"("data[0]"=w260) -> ("日期/时间字符串"=w259:string)  [unwired: 10 in]
                            n232 = call "数据编码.vi"("table输入"="实时数据" ("新元素/子数组"), "QN"=w248, "MN"=w256, "PW"=w255) -> ("错误常量"=w254:errorcluster, "通讯包字符串"=w258:string)  [unwired: 10 in]
                            n233 = global write "全局 时间2.vi" "加标回收索引起始时间"(w259) -> ()
                            n234 = global write "全局1.vi" "发送报文显示"(w258) -> ()
                            n235 = call "通信状态入队列.vi"("错误输入（无错误）"=w254, "枚举"=enum16{"打开连接", "发送数据", "读取数据", "数据处理", "关闭连接"}."发送数据") -> ()  [unwired: 9 in, 1 out]
                            n236 = Wait (ms)(milliseconds to wait=u32 1000 ("等待时间（毫秒）")) -> ()  [unwired: 1 out]
                          }
                        }
                      }
                    }
                    frame True {
                    }
                  }
                }
              }
            }
            frame "平行样" {
              n237 = flat-sequence {
                tunnel: [T2."集成干预"] -> w267
                frame #0 {
                  n238 = global write "全局 小时数据发送次数.vi" "小时数据发送次数"(0 ("小时数据发送次数")) -> ()
                  n239 = global write "全局 实时数据参数.vi" "实时数据参数"("平行样测试") -> ()
                  n240 = global write "全局1.vi" "枚举"(enum16{"返回请求应答", "上传数据", "返回执行结果"}."上传数据" ("枚举")) -> ()
                }
                frame #1 {
                  (unwired) "e" ("列队名（唯一）")
                  n241 = call "从数据库获取数据通用可配置(子VI).vi"("table输入"="平行样测试" ("新元素/子数组")) -> ()  [unwired: 9 in, 2 out]
                }
                frame #2 {
                  n242 = global read "全局 数据发送重叠.vi" "掉线指示灯"() -> (w273:bool)
                  n243 = Not(x=w273) -> (.not. x?=w272:bool)
                  n244 = case shown="真" w272 {
                    frame False {
                    }
                    frame True {
                      n245 = global read "全局 时间2.vi" "平行样索引"() -> (w277:T11)
                      n246 = Cluster To Array(cluster=w277) -> (array=w276:string[])
                      n247 = for {
                        tunnel: [w279] -> w274 mode=indexing
                        tunnel: w276 -> [w278] mode=indexing
                        i -> [w280]
                        # "行数大于零"
                        n248 = case shown="4" w280 {
                          tunnel: [w285 w286 w287 w288 w289] -> w281
                          frame 0, Default {
                            n249 = global read "全局 所有参数.vi" "氨氮"() -> (w285:string[][])
                          }
                          frame 1 {
                            n250 = global read "全局 所有参数.vi" "总磷"() -> (w286:string[][])
                          }
                          frame 2 {
                            n251 = global read "全局 所有参数.vi" "总氮"() -> (w287:string[][])
                          }
                          frame 3 {
                            n252 = global read "全局 所有参数.vi" "CODMn"() -> (w288:string[][])
                          }
                          frame 4 {
                            n253 = global read "全局 所有参数.vi" "CODCr"() -> (w289:string[][])
                          }
                        }
                        n254 = Array Size(array=w281) -> (size(s)=w283:i32[])
                        n255 = Index Array(array=w283) -> (element=w282:i32)  [unwired: 1 in]
                        n256 = Greater Than 0?(x=w282) -> (x > 0?=w284:bool)
                        n257 = case shown="真" w284 {
                          tunnel: w280 -> [_ _]
                          tunnel: w282 -> [_ _]
                          tunnel: w281 -> [_ w294]
                          tunnel: [w290 w291] -> w279
                          tunnel: w278 -> [w290 _]
                          frame False {
                          }
                          frame True {
                            # "最新时间戳加1分钟"
                            n258 = Array Size(array=w294) -> (size(s)=w296:i32[])
                            n259 = Index Array(array=w296) -> (element=w295:i32)  [unwired: 1 in]
                            n260 = Decrement(x=w295) -> (x-1=w293:i32)
                            n261 = Index Array(array=w294, index (row)=w293, index (col)=0 ("禁用的索引 (列)")) -> (element=w297:string)
                            n262 = call "日期时间字符串转换分钟数加一.vi"("data[0]"=w297) -> ("日期/时间字符串"=w291:string)  [unwired: 10 in]
                          }
                        }
                      }
                      n263 = Array To Cluster(array=w274) -> (cluster=w275:T10)
                      n264 = global write "全局 时间2.vi" "平行样索引"(w275) -> ()
                    }
                  }
                }
                frame #3 {
                  n265 = call "数据处理整合 (子VI).vi"("枚举"=enum16{"实时数据排序", "小时数据排序"}."实时数据排序") -> ("已排序的数组"=w300:string[])  [unwired: 10 in]
                  n266 = Array Size(array=w300) -> (size(s)=w299:i32)
                  n267 = global write "全局 数据数组大小.vi" "数据数组大小"(w299) -> ()
                }
                frame #4 {
                  n268 = global read "全局 数据发送重叠.vi" "掉线指示灯"() -> (w301:bool)
                  n269 = case shown="假" w301 {
                    frame False {
                      n270 = global read "全局 数据数组大小.vi" "数据数组大小"() -> (w303:i32)
                      n271 = Greater Than 0?(x=w303) -> (x > 0?=w304:bool)
                      n272 = case shown="真" w304 {
                        tunnel: w303 -> [_ w305]
                        frame False {
                        }
                        frame True {
                          n273 = for {
                            N: w305 -> [_]
                            i -> [w306]
                            n274 = Get Date/Time In Seconds() -> (seconds since 1Jan1904=w310:timestamp)
                            n275 = global write "全局 小时数据发送次数.vi" "小时数据发送次数"(w306) -> ()
                            n276 = Format Date/Time String(time format string (%c)="%Y%m%d%H%M%S%3u" ("时间格式字符串(%c)"), seconds (now)=w310) -> (date/time string=w309:string)  [unwired: 1 in]
                            n277 = Search and Replace String(input string=w309, search string="." ("搜索字符串")) -> (result string=w307:string)  [unwired: 6 in, 3 out]
                            n278 = global read "断电保存全局.vi" "MN"() -> (w315:string)
                            n279 = global read "断电保存全局.vi" "PW"() -> (w314:string)
                            n280 = call "数据编码.vi"("table输入"="实时数据" ("新元素/子数组"), "QN"=w307, "MN"=w315, "PW"=w314) -> ("错误常量"=w313:errorcluster, "通讯包字符串"=w317:string)  [unwired: 10 in]
                            n281 = global write "全局1.vi" "发送报文显示"(w317) -> ()
                            n282 = call "通信状态入队列.vi"("错误输入（无错误）"=w313, "枚举"=enum16{"打开连接", "发送数据", "读取数据", "数据处理", "关闭连接"}."发送数据") -> ()  [unwired: 9 in, 1 out]
                            n283 = Wait (ms)(milliseconds to wait=u32 1000 ("等待时间（毫秒）")) -> ()  [unwired: 1 out]
                          }
                        }
                      }
                    }
                    frame True {
                    }
                  }
                }
              }
            }
            frame "集成干预" {
              n284 = flat-sequence {
                tunnel: [T2."集成干预"] -> w319
                frame #0 {
                  n285 = global write "全局 小时数据发送次数.vi" "小时数据发送次数"(0 ("小时数据发送次数")) -> ()
                  n286 = global write "全局 实时数据参数.vi" "实时数据参数"("集成干预测试") -> ()
                  n287 = global write "全局1.vi" "枚举"(enum16{"返回请求应答", "上传数据", "返回执行结果"}."上传数据" ("枚举")) -> ()
                }
                frame #1 {
                  (unwired) "f" ("列队名（唯一）")
                  n288 = call "从数据库获取数据通用可配置(子VI).vi"("table输入"="集成干预测试" ("新元素/子数组")) -> ()  [unwired: 9 in, 2 out]
                }
                frame #2 {
                  n289 = global read "全局 数据发送重叠.vi" "掉线指示灯"() -> (w326:bool)
                  n290 = Not(x=w326) -> (.not. x?=w325:bool)
                  n291 = case shown="真" w325 {
                    frame False {
                    }
                    frame True {
                      n292 = global read "全局 时间2.vi" "集成干预索引"() -> (w330:T12)
                      n293 = Cluster To Array(cluster=w330) -> (array=w329:string[])
                      n294 = for {
                        tunnel: [w332] -> w327 mode=indexing
                        tunnel: w329 -> [w331] mode=indexing
                        i -> [w333]
                        # "行数大于零"
                        n295 = case shown="0, 默认" w333 {
                          tunnel: [w338 w339 w340 w341 w342 w343 w344 w345 w346 w347 w348 w349 w350 w351 w352] -> w334
                          frame 0, Default {
                            n296 = global read "全局 所有参数.vi" "氨氮"() -> (w338:string[][])
                          }
                          frame 1 {
                            n297 = global read "全局 所有参数.vi" "总磷"() -> (w339:string[][])
                          }
                          frame 2 {
                            n298 = global read "全局 所有参数.vi" "总氮"() -> (w340:string[][])
                          }
                          frame 3 {
                            n299 = global read "全局 所有参数.vi" "CODMn"() -> (w341:string[][])
                          }
                          frame 4 {
                            n300 = global read "全局 所有参数.vi" "CODCr"() -> (w342:string[][])
                          }
                          frame 5 {
                            n301 = global read "全局 所有参数.vi" "DO"() -> (w343:string[][])
                          }
                          frame 6 {
                            n302 = global read "全局 所有参数.vi" "PH"() -> (w344:string[][])
                          }
                          frame 7 {
                            n303 = global read "全局 所有参数.vi" "电导率"() -> (w345:string[][])
                          }
                          frame 8 {
                            n304 = global read "全局 所有参数.vi" "水温"() -> (w346:string[][])
                          }
                          frame 9 {
                            n305 = global read "全局 所有参数.vi" "浊度"() -> (w347:string[][])
                          }
                          frame 10 {
                            n306 = global read "全局 所有参数.vi" "叶绿素"() -> (w348:string[][])
                          }
                          frame 11 {
                            n307 = global read "全局 所有参数.vi" "藻密度"() -> (w349:string[][])
                          }
                          frame 12 {
                            n308 = global read "全局 所有参数.vi" "亚硝酸盐"() -> (w350:string[][])
                          }
                          frame 13 {
                            n309 = global read "全局 所有参数.vi" "硫化物"() -> (w351:string[][])
                          }
                          frame 14 {
                            n310 = global read "全局 所有参数.vi" "ORP"() -> (w352:string[][])
                          }
                        }
                        n311 = Array Size(array=w334) -> (size(s)=w336:i32[])
                        n312 = Index Array(array=w336) -> (element=w335:i32)  [unwired: 1 in]
                        n313 = Greater Than 0?(x=w335) -> (x > 0?=w337:bool)
                        n314 = case shown="真" w337 {
                          tunnel: w333 -> [_ _]
                          tunnel: w335 -> [_ _]
                          tunnel: w334 -> [_ w355]
                          tunnel: [w353 w354] -> w332
                          tunnel: w331 -> [w353 _]
                          frame False {
                          }
                          frame True {
                            # "最新时间戳加1分钟"
                            n315 = Array Size(array=w355) -> (size(s)=w359:i32[])
                            n316 = Index Array(array=w359) -> (element=w358:i32)  [unwired: 1 in]
                            n317 = Decrement(x=w358) -> (x-1=w357:i32)
                            n318 = Index Array(array=w355, index (row)=w357, index (col)=0 ("禁用的索引 (列)")) -> (element=w360:string)
                            n319 = call "日期时间字符串转换分钟数加一.vi"("data[0]"=w360) -> ("日期/时间字符串"=w354:string)  [unwired: 10 in]
                          }
                        }
                      }
                      n320 = Array To Cluster(array=w327) -> (cluster=w328:T8)
                      n321 = global write "全局 时间2.vi" "集成干预索引"(w328) -> ()
                    }
                  }
                }
                frame #3 {
                  n322 = call "数据处理整合 (子VI).vi"("枚举"=enum16{"实时数据排序", "小时数据排序"}."实时数据排序") -> ("已排序的数组"=w363:string[])  [unwired: 10 in]
                  n323 = Array Size(array=w363) -> (size(s)=w362:i32)
                  n324 = global write "全局 数据数组大小.vi" "数据数组大小"(w362) -> ()
                }
                frame #4 {
                  n325 = global read "全局 数据发送重叠.vi" "掉线指示灯"() -> (w365:bool)
                  n326 = case shown="假" w365 {
                    frame False {
                      n327 = global read "全局 数据数组大小.vi" "数据数组大小"() -> (w366:i32)
                      n328 = Greater Than 0?(x=w366) -> (x > 0?=w367:bool)
                      n329 = case shown="真" w367 {
                        tunnel: w366 -> [_ w368]
                        frame False {
                        }
                        frame True {
                          n330 = for {
                            N: w368 -> [_]
                            i -> [w369]
                            n331 = Get Date/Time In Seconds() -> (seconds since 1Jan1904=w373:timestamp)
                            n332 = Format Date/Time String(time format string (%c)="%Y%m%d%H%M%S%3u" ("时间格式字符串(%c)"), seconds (now)=w373) -> (date/time string=w372:string)  [unwired: 1 in]
                            n333 = global write "全局 小时数据发送次数.vi" "小时数据发送次数"(w369) -> ()
                            n334 = global read "断电保存全局.vi" "MN"() -> (w377:string)
                            n335 = global read "断电保存全局.vi" "PW"() -> (w376:string)
                            n336 = Search and Replace String(input string=w372, search string="." ("搜索字符串")) -> (result string=w370:string)  [unwired: 6 in, 3 out]
                            n337 = call "数据编码.vi"("table输入"="实时数据" ("新元素/子数组"), "QN"=w370, "MN"=w377, "PW"=w376) -> ("错误常量"=w378:errorcluster, "通讯包字符串"=w380:string)  [unwired: 10 in]
                            n338 = global write "全局1.vi" "发送报文显示"(w380) -> ()
                            n339 = call "通信状态入队列.vi"("错误输入（无错误）"=w378, "枚举"=enum16{"打开连接", "发送数据", "读取数据", "数据处理", "关闭连接"}."发送数据") -> ()  [unwired: 9 in, 1 out]
                            n340 = Wait (ms)(milliseconds to wait=u32 1000 ("等待时间（毫秒）")) -> ()  [unwired: 1 out]
                          }
                        }
                      }
                    }
                    frame True {
                    }
                  }
                }
              }
            }
          }
        }
      }
      frame "操作日志" {
        # "间隔时间上传"
        # "直接1分钟查询 一次,有数据就按数据上传,没数据就不上传,在数据发送那边有做处理"
        n341 = flat-sequence {
          frame #0 {
            # "时间"
            n342 = global write "全局 小时数据发送次数.vi" "小时数据发送次数"(0 ("小时数据发送次数")) -> ()
            n343 = call "日志信息主动发送(子VI).vi"() -> ()  [unwired: 12 in]
            n344 = global write "全局1.vi" "枚举"(enum16{"返回请求应答", "上传数据", "返回执行结果"}."上传数据" ("枚举")) -> ()
          }
          frame #1 {
            n345 = call "获取操作日志 (子VI).vi"("table输入"="操作日志") -> ()  [unwired: 11 in]
          }
          frame #2 {
            n346 = global read "全局 数据发送重叠.vi" "掉线指示灯"() -> (w387:bool)
            n347 = Not(x=w387) -> (.not. x?=w386:bool)
            n348 = case shown="真" w386 {
              frame False {
              }
              frame True {
                n349 = global read "全局 时间2.vi" "仪器日志索引"() -> (w391:T13)
                n350 = Cluster To Array(cluster=w391) -> (array=w390:string[])
                n351 = for {
                  tunnel: w390 -> [w392] mode=indexing
                  tunnel: [w393] -> w388 mode=indexing
                  i -> [w395]
                  # "行数大于零"
                  n352 = case shown="5" w395 {
                    tunnel: [w399 w400 w401 w402 w403 w404] -> w394
                    frame 0, Default {
                      n353 = global read "全局 所有参数.vi" "氨氮"() -> (w399:string[][])
                    }
                    frame 1 {
                      n354 = global read "全局 所有参数.vi" "总磷"() -> (w400:string[][])
                    }
                    frame 2 {
                      n355 = global read "全局 所有参数.vi" "总氮"() -> (w401:string[][])
                    }
                    frame 3 {
                      n356 = global read "全局 所有参数.vi" "CODMn"() -> (w402:string[][])
                    }
                    frame 4 {
                      n357 = global read "全局 所有参数.vi" "CODCr"() -> (w403:string[][])
                    }
                    frame 5 {
                      n358 = global read "全局 所有参数.vi" "DO"() -> (w404:string[][])
                    }
                  }
                  n359 = Array Size(array=w394) -> (size(s)=w397:i32[])
                  n360 = Index Array(array=w397) -> (element=w396:i32)  [unwired: 1 in]
                  n361 = Greater Than 0?(x=w396) -> (x > 0?=w398:bool)
                  n362 = case shown="真" w398 {
                    tunnel: w396 -> [_ _]
                    tunnel: w394 -> [_ w410]
                    tunnel: [w405 w406] -> w393
                    tunnel: w392 -> [w405 _]
                    frame False {
                    }
                    frame True {
                      # "最新时间戳加1分钟"
                      n363 = Array Size(array=w410) -> (size(s)=w412:i32[])
                      n364 = Index Array(array=w412) -> (element=w411:i32)  [unwired: 1 in]
                      n365 = Decrement(x=w411) -> (x-1=w409:i32)
                      n366 = Index Array(array=w410, index (row)=w409, index (col)=0 ("禁用的索引 (列)")) -> (element=w407:string)
                      n367 = call "日期时间字符串转换秒数加一.vi"("data[0]"=w407) -> ("日期/时间字符串"=w406:string)  [unwired: 10 in]
                    }
                  }
                }
                n368 = Array To Cluster(array=w388) -> (cluster=w389:T14)
                n369 = global write "全局 时间2.vi" "仪器日志索引"(w389) -> ()
              }
            }
          }
          frame #3 {
            n370 = call "数据处理整合 (子VI).vi"("枚举"=enum16{"实时数据排序", "小时数据排序"}."实时数据排序") -> ("已排序的数组"=w415:string[])  [unwired: 10 in]
            n371 = Array Size(array=w415) -> (size(s)=w414:i32)
            n372 = global write "全局 数据数组大小.vi" "数据数组大小"(w414) -> ()
          }
          frame #4 {
            # "判定是否存表"
            n373 = global read "全局 数据发送重叠.vi" "掉线指示灯"() -> (w416:bool)
            n374 = case shown="假" w416 {
              frame False {
                n375 = global read "全局 数据数组大小.vi" "数据数组大小"() -> (w417:i32)
                n376 = Greater Than 0?(x=w417) -> (x > 0?=w418:bool)
                n377 = case shown="真" w418 {
                  frame False {
                  }
                  frame True {
                    n378 = while {
                      stop <- w420 stop-if-true
                      n379 = Get Date/Time In Seconds() -> (seconds since 1Jan1904=w432:timestamp)
                      n380 = Format Date/Time String(time format string (%c)="%Y%m%d%H%M%S%3u" ("时间格式字符串(%c)"), seconds (now)=w432) -> (date/time string=w431:string)  [unwired: 1 in]
                      n381 = Search and Replace String(input string=w431, search string="." ("搜索字符串")) -> (result string=w429:string)  [unwired: 6 in, 3 out]
                      n382 = global read "断电保存全局.vi" "MN"() -> (w426:string)
                      n383 = global read "断电保存全局.vi" "PW"() -> (w425:string)
                      n384 = call "数据编码.vi"("table输入"="操作日志" ("新元素/子数组"), "QN"=w429, "MN"=w426, "PW"=w425) -> ("错误常量"=w424:errorcluster, "通讯包字符串"=w428:string)  [unwired: 10 in]
                      n385 = global read "全局 小时数据发送次数.vi" "小时数据发送次数"() -> (w421:i32)
                      n386 = global read "全局 数据数组大小.vi" "数据数组大小"() -> (w422:i32)
                      n387 = call "通信状态入队列.vi"("错误输入（无错误）"=w424, "枚举"=enum16{"打开连接", "发送数据", "读取数据", "数据处理", "关闭连接"}."发送数据") -> ()  [unwired: 9 in, 1 out]
                      n388 = global write "全局1.vi" "发送报文显示"(w428) -> ()
                      n389 = Decrement(x=w422) -> (x-1=w423:i32)
                      n390 = Greater Or Equal?(x=w421, y=w423) -> (x >= y?=w420:bool)
                      n391 = Wait (ms)(milliseconds to wait=u32 1000 ("等待时间（毫秒）")) -> ()  [unwired: 1 out]
                    }
                  }
                }
              }
              frame True {
              }
            }
          }
        }
      }
      frame "仪器参数" {
        # "间隔时间上传"
        # "直接1分钟查询 一次,有数据就按数据上传,没数据就不上传,在数据发送那边有做处理"
        n392 = flat-sequence {
          frame #0 {
            n393 = global write "全局 小时数据发送次数.vi" "小时数据发送次数"(0 ("小时数据发送次数")) -> ()
            n394 = global write "全局1.vi" "枚举"(enum16{"返回请求应答", "上传数据", "返回执行结果"}."上传数据" ("枚举")) -> ()
          }
          frame #1 {
            n395 = call "获取操作日志 (子VI).vi"("table输入"="仪器参数") -> ()  [unwired: 11 in]
          }
          frame #2 {
            n396 = global read "全局 数据发送重叠.vi" "掉线指示灯"() -> (w440:bool)
            n397 = Not(x=w440) -> (.not. x?=w439:bool)
            n398 = case shown="真" w439 {
              frame False {
              }
              frame True {
                n399 = global read "全局 时间2.vi" "仪器参数索引"() -> (w444:T15)
                n400 = Cluster To Array(cluster=w444) -> (array=w443:string[])
                n401 = for {
                  tunnel: [w448] -> w441 mode=indexing
                  tunnel: w443 -> [w447] mode=indexing
                  i -> [w446]
                  # "行数大于零"
                  n402 = case shown="12" w446 {
                    tunnel: [w452 w453 w454 w455 w456 w457 w458 w459 w460 w461 w462 w463 w464] -> w445
                    frame 0, Default {
                      n403 = global read "全局 所有参数.vi" "氨氮"() -> (w452:string[][])
                    }
                    frame 1 {
                      n404 = global read "全局 所有参数.vi" "总磷"() -> (w453:string[][])
                    }
                    frame 2 {
                      n405 = global read "全局 所有参数.vi" "总氮"() -> (w454:string[][])
                    }
                    frame 3 {
                      n406 = global read "全局 所有参数.vi" "CODMn"() -> (w455:string[][])
                    }
                    frame 4 {
                      n407 = global read "全局 所有参数.vi" "CODCr"() -> (w456:string[][])
                    }
                    frame 5 {
                      n408 = global read "全局 所有参数.vi" "DO"() -> (w457:string[][])
                    }
                    frame 6 {
                      n409 = global read "全局 所有参数.vi" "PH"() -> (w458:string[][])
                    }
                    frame 7 {
                      n410 = global read "全局 所有参数.vi" "电导率"() -> (w459:string[][])
                    }
                    frame 8 {
                      n411 = global read "全局 所有参数.vi" "水温"() -> (w460:string[][])
                    }
                    frame 9 {
                      n412 = global read "全局 所有参数.vi" "浊度"() -> (w461:string[][])
                    }
                    frame 10 {
                      n413 = global read "全局 所有参数.vi" "叶绿素"() -> (w462:string[][])
                    }
                    frame 11 {
                      n414 = global read "全局 所有参数.vi" "藻密度"() -> (w463:string[][])
                    }
                    frame 12 {
                      n415 = global read "全局 所有参数.vi" "ORP"() -> (w464:string[][])
                    }
                  }
                  n416 = Array Size(array=w445) -> (size(s)=w450:i32[])
                  n417 = Index Array(array=w450) -> (element=w449:i32)  [unwired: 1 in]
                  n418 = Greater Than 0?(x=w449) -> (x > 0?=w451:bool)
                  n419 = case shown="真" w451 {
                    tunnel: w449 -> [_ _]
                    tunnel: w445 -> [_ w469]
                    tunnel: [w465 w466] -> w448
                    tunnel: w447 -> [w465 _]
                    frame False {
                    }
                    frame True {
                      # "最新时间戳加1分钟"
                      n420 = Array Size(array=w469) -> (size(s)=w471:i32[])
                      n421 = Index Array(array=w471) -> (element=w470:i32)  [unwired: 1 in]
                      n422 = Decrement(x=w470) -> (x-1=w468:i32)
                      n423 = Index Array(array=w469, index (row)=w468, index (col)=0 ("禁用的索引 (列)")) -> (element=w472:string)
                      n424 = call "日期时间字符串转换分钟数加一.vi"("data[0]"=w472) -> ("日期/时间字符串"=w466:string)  [unwired: 10 in]
                    }
                  }
                }
                n425 = Array To Cluster(array=w441) -> (cluster=w442:T16)
                n426 = global write "全局 时间2.vi" "仪器参数索引"(w442) -> ()
              }
            }
          }
          frame #3 {
            n427 = call "数据处理整合 (子VI).vi"("枚举"=enum16{"实时数据排序", "小时数据排序"}."实时数据排序") -> ("已排序的数组"=w475:string[])  [unwired: 10 in]
            n428 = Array Size(array=w475) -> (size(s)=w474:i32)
            n429 = global write "全局 数据数组大小.vi" "数据数组大小"(w474) -> ()
          }
          frame #4 {
            # "判定是否存表"
            n430 = global read "全局 数据发送重叠.vi" "掉线指示灯"() -> (w476:bool)
            n431 = case shown="假" w476 {
              frame False {
                n432 = global read "全局 数据数组大小.vi" "数据数组大小"() -> (w477:i32)
                n433 = Greater Than 0?(x=w477) -> (x > 0?=w478:bool)
                n434 = case shown="真" w478 {
                  frame False {
                  }
                  frame True {
                    n435 = while {
                      stop <- w479 stop-if-true
                      n436 = Get Date/Time In Seconds() -> (seconds since 1Jan1904=w492:timestamp)
                      n437 = Format Date/Time String(time format string (%c)="%Y%m%d%H%M%S%3u" ("时间格式字符串(%c)"), seconds (now)=w492) -> (date/time string=w491:string)  [unwired: 1 in]
                      n438 = Search and Replace String(input string=w491, search string="." ("搜索字符串")) -> (result string=w489:string)  [unwired: 6 in, 3 out]
                      n439 = global read "断电保存全局.vi" "MN"() -> (w486:string)
                      n440 = global read "断电保存全局.vi" "PW"() -> (w485:string)
                      n441 = global read "全局 数据数组大小.vi" "数据数组大小"() -> (w481:i32)
                      n442 = call "数据编码.vi"("table输入"="仪器参数" ("新元素/子数组"), "QN"=w489, "MN"=w486, "PW"=w485) -> ("错误常量"=w484:errorcluster, "通讯包字符串"=w488:string)  [unwired: 10 in]
                      n443 = global read "全局 小时数据发送次数.vi" "小时数据发送次数"() -> (w482:i32)
                      n444 = global write "全局1.vi" "发送报文显示"(w488) -> ()
                      n445 = call "通信状态入队列.vi"("错误输入（无错误）"=w484, "枚举"=enum16{"打开连接", "发送数据", "读取数据", "数据处理", "关闭连接"}."发送数据") -> ()  [unwired: 9 in, 1 out]
                      n446 = Decrement(x=w481) -> (x-1=w480:i32)
                      n447 = Greater Or Equal?(x=w482, y=w480) -> (x >= y?=w479:bool)
                      n448 = Wait (ms)(milliseconds to wait=u32 1000 ("等待时间（毫秒）")) -> ()  [unwired: 1 out]
                    }
                  }
                }
              }
              frame True {
              }
            }
          }
        }
      }
      frame "系统状态" {
        # "直接1分钟查询 一次,有变化就按上传,没变化就不上传"
        n449 = flat-sequence {
          frame #0 {
            # "时间"
            n450 = global write "全局 小时数据发送次数.vi" "小时数据发送次数"(0 ("小时数据发送次数")) -> ()
            n451 = global write "全局 数据数组大小.vi" "数据数组大小"(1 ("数据数组大小")) -> ()
            n452 = global write "全局1.vi" "枚举"(enum16{"返回请求应答", "上传数据", "返回执行结果"}."上传数据" ("枚举")) -> ()
          }
          frame #1 {
            # "判定是否存表"
            n453 = global read "全局 数据发送重叠.vi" "掉线指示灯"() -> (w499:bool)
            n454 = case shown="假" w499 {
              frame False {
                n455 = global read "全局1.vi" "系统状态"() -> (w500:bool)
                n456 = case shown="真" w500 {
                  frame False {
                  }
                  frame True {
                    n457 = global read "全局 小时数据发送次数.vi" "小时数据发送次数"() -> (w508:i32)
                    n458 = global write "全局1.vi" "系统状态"(FALSE ("系统状态")) -> ()
                    n459 = Get Date/Time In Seconds() -> (seconds since 1Jan1904=w512:timestamp)
                    n460 = Increment(x=w508) -> (x+1=w507:i32)
                    n461 = Format Date/Time String(time format string (%c)="%Y%m%d%H%M%S%3u" ("时间格式字符串(%c)"), seconds (now)=w512) -> (date/time string=w511:string)  [unwired: 1 in]
                    n462 = global write "全局 小时数据发送次数.vi" "小时数据发送次数"(w507) -> ()
                    n463 = Search and Replace String(input string=w511, search string="." ("搜索字符串")) -> (result string=w509:string)  [unwired: 6 in, 3 out]
                    n464 = global read "断电保存全局.vi" "MN"() -> (w504:string)
                    n465 = global read "断电保存全局.vi" "PW"() -> (w503:string)
                    n466 = call "数据编码.vi"("table输入"="系统状态" ("新元素/子数组"), "QN"=w509, "MN"=w504, "PW"=w503) -> ("错误常量"=w502:errorcluster, "通讯包字符串"=w506:string)  [unwired: 10 in]
                    n467 = call "通信状态入队列.vi"("错误输入（无错误）"=w502, "枚举"=enum16{"打开连接", "发送数据", "读取数据", "数据处理", "关闭连接"}."发送数据") -> ()  [unwired: 9 in, 1 out]
                    n468 = global write "全局1.vi" "发送报文显示"(w506) -> ()
                  }
                }
              }
              frame True {
              }
            }
          }
        }
      }
      frame "运行模式" {
        # "直接1分钟查询 一次,有变化就按上传,没变化就不上传"
        n469 = flat-sequence {
          frame #0 {
            # "时间"
            n470 = global write "全局 小时数据发送次数.vi" "小时数据发送次数"(0 ("小时数据发送次数")) -> ()
            n471 = global write "全局 数据数组大小.vi" "数据数组大小"(1 ("数据数组大小")) -> ()
            n472 = global write "全局1.vi" "枚举"(enum16{"返回请求应答", "上传数据", "返回执行结果"}."上传数据" ("枚举")) -> ()
          }
          frame #1 {
            # "判定是否存表"
            n473 = global read "全局 数据发送重叠.vi" "掉线指示灯"() -> (w519:bool)
            n474 = case shown="假" w519 {
              frame False {
                n475 = global read "全局1.vi" "运行模式"() -> (w520:bool)
                n476 = case shown="真" w520 {
                  frame False {
                  }
                  frame True {
                    n477 = global read "全局 小时数据发送次数.vi" "小时数据发送次数"() -> (w528:i32)
                    n478 = global write "全局1.vi" "运行模式"(FALSE ("系统状态")) -> ()
                    n479 = Get Date/Time In Seconds() -> (seconds since 1Jan1904=w532:timestamp)
                    n480 = Increment(x=w528) -> (x+1=w527:i32)
                    n481 = Format Date/Time String(time format string (%c)="%Y%m%d%H%M%S%3u" ("时间格式字符串(%c)"), seconds (now)=w532) -> (date/time string=w531:string)  [unwired: 1 in]
                    n482 = global write "全局 小时数据发送次数.vi" "小时数据发送次数"(w527) -> ()
                    n483 = Search and Replace String(input string=w531, search string="." ("搜索字符串")) -> (result string=w529:string)  [unwired: 6 in, 3 out]
                    n484 = global read "断电保存全局.vi" "MN"() -> (w524:string)
                    n485 = global read "断电保存全局.vi" "PW"() -> (w523:string)
                    n486 = call "数据编码.vi"("table输入"="运行模式" ("新元素/子数组"), "QN"=w529, "MN"=w524, "PW"=w523) -> ("错误常量"=w522:errorcluster, "通讯包字符串"=w526:string)  [unwired: 10 in]
                    n487 = call "通信状态入队列.vi"("错误输入（无错误）"=w522, "枚举"=enum16{"打开连接", "发送数据", "读取数据", "数据处理", "关闭连接"}."发送数据") -> ()  [unwired: 9 in, 1 out]
                    n488 = global write "全局1.vi" "发送报文显示"(w526) -> ()
                  }
                }
              }
              frame True {
              }
            }
          }
        }
      }
      frame "测量周期" {
        # "直接1分钟查询 一次,有变化就按上传,没变化就不上传"
        n489 = flat-sequence {
          frame #0 {
            # "时间"
            n490 = global write "全局 小时数据发送次数.vi" "小时数据发送次数"(0 ("小时数据发送次数")) -> ()
            n491 = global write "全局 数据数组大小.vi" "数据数组大小"(1 ("数据数组大小")) -> ()
            n492 = global write "全局1.vi" "枚举"(enum16{"返回请求应答", "上传数据", "返回执行结果"}."上传数据" ("枚举")) -> ()
          }
          frame #1 {
            # "判定是否存表"
            n493 = global read "全局 数据发送重叠.vi" "掉线指示灯"() -> (w539:bool)
            n494 = case shown="假" w539 {
              frame False {
                n495 = global read "全局1.vi" "测量周期"() -> (w540:bool)
                n496 = case shown="真" w540 {
                  frame False {
                  }
                  frame True {
                    n497 = global read "全局 小时数据发送次数.vi" "小时数据发送次数"() -> (w548:i32)
                    n498 = global write "全局1.vi" "测量周期"(FALSE ("系统状态")) -> ()
                    n499 = Get Date/Time In Seconds() -> (seconds since 1Jan1904=w552:timestamp)
                    n500 = Increment(x=w548) -> (x+1=w547:i32)
                    n501 = Format Date/Time String(time format string (%c)="%Y%m%d%H%M%S%3u" ("时间格式字符串(%c)"), seconds (now)=w552) -> (date/time string=w551:string)  [unwired: 1 in]
                    n502 = global write "全局 小时数据发送次数.vi" "小时数据发送次数"(w547) -> ()
                    n503 = Search and Replace String(input string=w551, search string="." ("搜索字符串")) -> (result string=w549:string)  [unwired: 6 in, 3 out]
                    n504 = global read "断电保存全局.vi" "MN"() -> (w544:string)
                    n505 = global read "断电保存全局.vi" "PW"() -> (w543:string)
                    n506 = call "数据编码.vi"("table输入"="测量周期" ("新元素/子数组"), "QN"=w549, "MN"=w544, "PW"=w543) -> ("错误常量"=w542:errorcluster, "通讯包字符串"=w546:string)  [unwired: 10 in]
                    n507 = global write "全局1.vi" "发送报文显示"(w546) -> ()
                    n508 = call "通信状态入队列.vi"("错误输入（无错误）"=w542, "枚举"=enum16{"打开连接", "发送数据", "读取数据", "数据处理", "关闭连接"}."发送数据") -> ()  [unwired: 9 in, 1 out]
                  }
                }
              }
              frame True {
              }
            }
          }
        }
      }
      frame "超标留样" {
        # "直接1分钟查询 一次,有变化就按上传,没变化就不上传"
        n509 = flat-sequence {
          frame #0 {
            # "时间"
            n510 = global write "全局 小时数据发送次数.vi" "小时数据发送次数"(0 ("小时数据发送次数")) -> ()
            n511 = global write "全局 数据数组大小.vi" "数据数组大小"(1 ("数据数组大小")) -> ()
            n512 = global write "全局1.vi" "枚举"(enum16{"返回请求应答", "上传数据", "返回执行结果"}."上传数据" ("枚举")) -> ()
          }
          frame #1 {
            # "判定是否存表"
            n513 = global read "全局 数据发送重叠.vi" "掉线指示灯"() -> (w559:bool)
            n514 = case shown="假" w559 {
              frame False {
                n515 = global read "全局1.vi" "超标留样"() -> (w560:bool)
                n516 = case shown="真" w560 {
                  frame False {
                  }
                  frame True {
                    n517 = global read "全局 小时数据发送次数.vi" "小时数据发送次数"() -> (w568:i32)
                    n518 = global write "全局1.vi" "超标留样"(FALSE ("系统状态")) -> ()
                    n519 = Get Date/Time In Seconds() -> (seconds since 1Jan1904=w572:timestamp)
                    n520 = Increment(x=w568) -> (x+1=w567:i32)
                    n521 = Format Date/Time String(time format string (%c)="%Y%m%d%H%M%S%3u" ("时间格式字符串(%c)"), seconds (now)=w572) -> (date/time string=w571:string)  [unwired: 1 in]
                    n522 = global write "全局 小时数据发送次数.vi" "小时数据发送次数"(w567) -> ()
                    n523 = Search and Replace String(input string=w571, search string="." ("搜索字符串")) -> (result string=w569:string)  [unwired: 6 in, 3 out]
                    n524 = global read "断电保存全局.vi" "MN"() -> (w563:string)
                    n525 = global read "断电保存全局.vi" "PW"() -> (w562:string)
                    n526 = call "数据编码.vi"("table输入"="超标留样" ("新元素/子数组"), "QN"=w569, "MN"=w563, "PW"=w562) -> ("错误常量"=w564:errorcluster, "通讯包字符串"=w566:string)  [unwired: 10 in]
                    n527 = global write "全局1.vi" "发送报文显示"(w566) -> ()
                    n528 = call "通信状态入队列.vi"("错误输入（无错误）"=w564, "枚举"=enum16{"打开连接", "发送数据", "读取数据", "数据处理", "关闭连接"}."发送数据") -> ()  [unwired: 9 in, 1 out]
                  }
                }
              }
              frame True {
              }
            }
          }
        }
      }
      frame "报警信息" {
        # "间隔时间上传"
        # "直接1分钟查询 一次,有数据就按数据上传,没数据为空的不传,在数据发送那边有做处理"
        n529 = flat-sequence {
          frame #0 {
            # "分钟时间间隔"
            n530 = call "日志信息主动发送(子VI).vi"() -> ()  [unwired: 12 in]
            n531 = global write "全局 小时数据发送次数.vi" "小时数据发送次数"(0 ("小时数据发送次数")) -> ()
            n532 = global write "全局1.vi" "枚举"(enum16{"返回请求应答", "上传数据", "返回执行结果"}."上传数据" ("枚举")) -> ()
          }
          frame #1 {
            n533 = call "获取报警信息 (子VI).vi"() -> ()  [unwired: 12 in]
          }
          frame #2 {
            n534 = global read "全局 数据发送重叠.vi" "掉线指示灯"() -> (w579:bool)
            n535 = Not(x=w579) -> (.not. x?=w578:bool)
            n536 = case shown="真" w578 {
              frame False {
              }
              frame True {
                n537 = global read "全局 时间2.vi" "报警信息索引"() -> (w583:T17)
                n538 = Cluster To Array(cluster=w583) -> (array=w582:string[])
                n539 = for {
                  tunnel: [w585] -> w580 mode=indexing
                  tunnel: w582 -> [w584] mode=indexing
                  i -> [w587]
                  # "行数大于零"
                  n540 = case shown="1" w587 {
                    tunnel: [w591 w592 w593 w594 w595 w596 w597 w598 w599 w600 w601 w602] -> w586
                    frame 0, Default {
                      n541 = global read "全局 所有参数.vi" "氨氮"() -> (w591:string[][])
                    }
                    frame 1 {
                      n542 = global read "全局 所有参数.vi" "总磷"() -> (w592:string[][])
                    }
                    frame 2 {
                      n543 = global read "全局 所有参数.vi" "总氮"() -> (w593:string[][])
                    }
                    frame 3 {
                      n544 = global read "全局 所有参数.vi" "CODMn"() -> (w594:string[][])
                    }
                    frame 4 {
                      n545 = global read "全局 所有参数.vi" "CODCr"() -> (w595:string[][])
                    }
                    frame 5 {
                      n546 = global read "全局 所有参数.vi" "DO"() -> (w596:string[][])
                    }
                    frame 6 {
                      n547 = global read "全局 所有参数.vi" "PH"() -> (w597:string[][])
                    }
                    frame 7 {
                      n548 = global read "全局 所有参数.vi" "电导率"() -> (w598:string[][])
                    }
                    frame 8 {
                      n549 = global read "全局 所有参数.vi" "水温"() -> (w599:string[][])
                    }
                    frame 9 {
                      n550 = global read "全局 所有参数.vi" "浊度"() -> (w600:string[][])
                    }
                    frame 10 {
                      n551 = global read "全局 所有参数.vi" "叶绿素"() -> (w601:string[][])
                    }
                    frame 11 {
                      n552 = global read "全局 所有参数.vi" "藻密度"() -> (w602:string[][])
                    }
                  }
                  n553 = Array Size(array=w586) -> (size(s)=w589:i32[])
                  n554 = Index Array(array=w589) -> (element=w588:i32)  [unwired: 1 in]
                  n555 = Greater Than 0?(x=w588) -> (x > 0?=w590:bool)
                  n556 = case shown="真" w590 {
                    tunnel: w588 -> [_ _]
                    tunnel: w586 -> [_ w607]
                    tunnel: [w603 w604] -> w585
                    tunnel: w584 -> [w603 _]
                    frame False {
                    }
                    frame True {
                      # "最新时间戳加1分钟"
                      n557 = Array Size(array=w607) -> (size(s)=w609:i32[])
                      n558 = Index Array(array=w609) -> (element=w608:i32)  [unwired: 1 in]
                      n559 = Decrement(x=w608) -> (x-1=w606:i32)
                      n560 = Index Array(array=w607, index (row)=w606, index (col)=0 ("禁用的索引 (列)")) -> (element=w610:string)
                      n561 = call "日期时间字符串转换分钟数加一.vi"("data[0]"=w610) -> ("日期/时间字符串"=w604:string)  [unwired: 10 in]
                    }
                  }
                }
                n562 = Array To Cluster(array=w580) -> (cluster=w581:T18)
                n563 = global write "全局 时间2.vi" "报警信息索引"(w581) -> ()
              }
            }
          }
          frame #3 {
            n564 = call "数据处理整合 (子VI).vi"("枚举"=enum16{"实时数据排序", "小时数据排序"}."实时数据排序") -> ("已排序的数组"=w613:string[])  [unwired: 10 in]
            n565 = Array Size(array=w613) -> (size(s)=w612:i32)
            n566 = global write "全局 数据数组大小.vi" "数据数组大小"(w612) -> ()
          }
          frame #4 {
            # "判定是否存表"
            n567 = global read "全局 数据发送重叠.vi" "掉线指示灯"() -> (w614:bool)
            n568 = case shown="假" w614 {
              frame False {
                # "判定数据不为空才发"
                n569 = global read "全局 数据数组大小.vi" "数据数组大小"() -> (w615:i32)
                n570 = Greater Than 0?(x=w615) -> (x > 0?=w616:bool)
                n571 = case shown="真" w616 {
                  frame False {
                    n572 = global write "全局1.vi" "核查数据上传"(FALSE ("数据上传")) -> ()
                  }
                  frame True {
                    n573 = while {
                      stop <- w619 stop-if-true
                      n574 = Wait (ms)(milliseconds to wait=u32 1000 ("等待时间（毫秒）")) -> ()  [unwired: 1 out]
                      n575 = Get Date/Time In Seconds() -> (seconds since 1Jan1904=w631:timestamp)
                      n576 = Format Date/Time String(time format string (%c)="%Y%m%d%H%M%S%3u" ("时间格式字符串(%c)"), seconds (now)=w631) -> (date/time string=w630:string)  [unwired: 1 in]
                      n577 = global read "全局 数据数组大小.vi" "数据数组大小"() -> (w621:i32)
                      n578 = Search and Replace String(input string=w630, search string="." ("搜索字符串")) -> (result string=w628:string)  [unwired: 6 in, 3 out]
                      n579 = global read "断电保存全局.vi" "MN"() -> (w625:string)
                      n580 = global read "断电保存全局.vi" "PW"() -> (w624:string)
                      n581 = global read "全局 小时数据发送次数.vi" "小时数据发送次数"() -> (w622:i32)
                      n582 = call "数据编码.vi"("table输入"="报警信息" ("新元素/子数组"), "QN"=w628, "MN"=w625, "PW"=w624) -> ("错误常量"=w623:errorcluster, "通讯包字符串"=w627:string)  [unwired: 10 in]
                      n583 = Decrement(x=w621) -> (x-1=w620:i32)
                      n584 = global write "全局1.vi" "发送报文显示"(w627) -> ()
                      n585 = Greater Or Equal?(x=w622, y=w620) -> (x >= y?=w619:bool)
                      n586 = call "通信状态入队列.vi"("错误输入（无错误）"=w623, "枚举"=enum16{"打开连接", "发送数据", "读取数据", "数据处理", "关闭连接"}."发送数据") -> ()  [unwired: 9 in, 1 out]
                    }
                  }
                }
              }
              frame True {
              }
            }
          }
        }
      }
      frame "环境参数" {
        n587 = call "核查数据断电保存 (子VI).vi"() -> ()  [unwired: 12 in]
      }
    }
    n588 = Not(x=w4) -> (.not. x?=w5:bool)
    n589 = global write "全局1.vi" "核查数据上传"(w5) -> ()
  }
  "错误输出" <- w1
